vi "Separate Inline and Async Plugins.vi"(8 "error in (no error)":errorcluster, 11 "Plugins":refnum<class "Plugin.lvclass">[](array[class])) -> (0 "error out":errorcluster, 2 "Async Plugins":refnum<class "Plugin.lvclass">[](array[class]), 3 "Inline Plugins":refnum<class "Plugin.lvclass">[](array[class]))   [LabVIEW 2017, in "DSF Core.lvlib" / "Plugin.lvclass"]
uses:
  Plugin/Plugin.lvclass
  Timing/Timing.lvclass
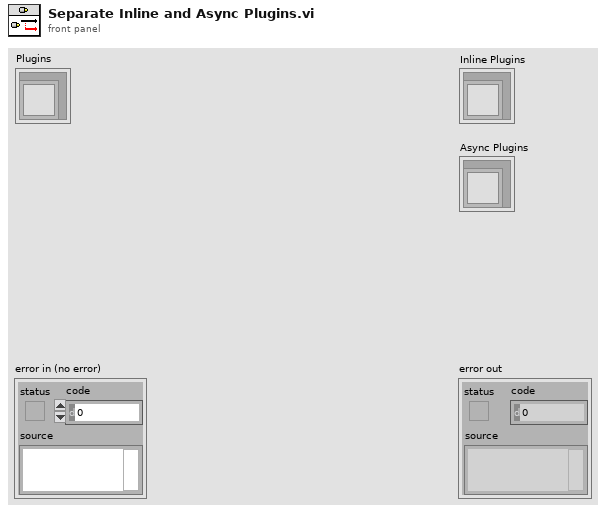
[diagram p1: front panel]
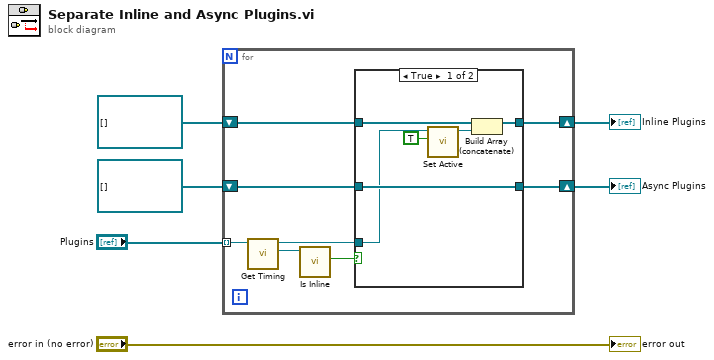
[diagram p0: block diagram]
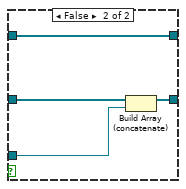
[diagram p2: hidden frame]
diagram:
  n1 = for {
    tunnel: "Plugins" -> [w14] mode=indexing
    shift-right: [w8] -> w2
    shift-left: refnum<class "Plugin.lvclass">[] [] ("Plugins 2") -> [w10]
    shift-right: [w7] -> w1
    shift-left: refnum<class "Plugin.lvclass">[] [] ("Plugins 2") -> [w9]
    n2 = call "Get Timing.vi"("Plugin in"=w14) -> ("Timing"=w13:refnum<class "Timing.lvclass">, "Plugin out"=w11:refnum<class "Plugin.lvclass">)  [unwired: 9 in]
    n3 = call "Is Inline.vi"("Timing in"=w13) -> ("inline?"=w12:bool)  [unwired: 9 in, 1 out]
    n4 = case shown="True" w12 {
      tunnel: w11 -> [w17 w21]
      tunnel: w10 -> [w20 w22]
      tunnel: w9 -> [w18 w24]
      tunnel: [w19 w22] -> w8
      tunnel: [w18 w23] -> w7
      frame True {
        n5 = call "Set Active.vi"("active"=TRUE, "Plugin in"=w17) -> ("Plugin out"=w16:refnum<class "Plugin.lvclass">)  [unwired: 9 in]
        n6 = Build Array (concatenate)(w20, w16) -> (w19:refnum<class "Plugin.lvclass">[])
      }
      frame False {
        n7 = Build Array (concatenate)(w24, w21) -> (w23:refnum<class "Plugin.lvclass">[])
      }
    }
  }
  "Inline Plugins" <- w2
  "Async Plugins" <- w1
  "error out" <- "error in (no error)"
